vi "AllAvrStdGraph.vi"() -> ()   [LabVIEW 2023]
panel:
  out "Numeric":dbl format="%#_4f"
  out "AvrSTDToArr - only six":dbl[](array[numeric]) format="%#_6f"
  out "Waveform Graph":dbl[][](graph)
  in  "const + StdAvr":dbl
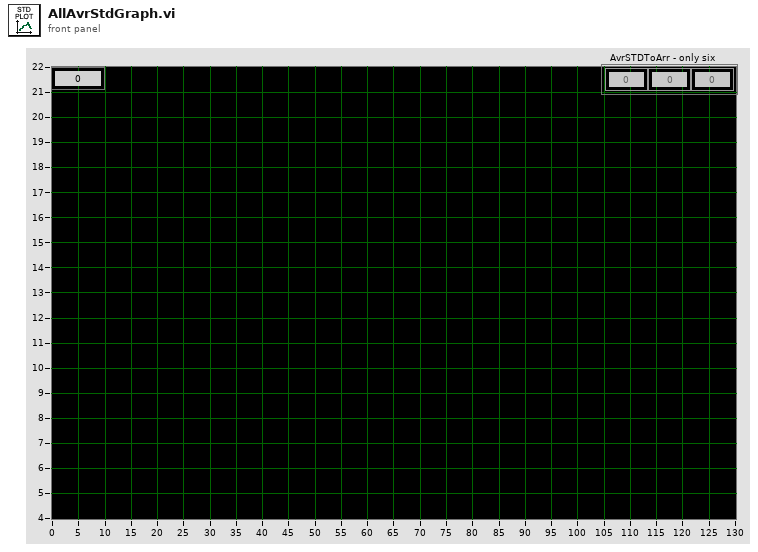
[diagram p1: front panel]
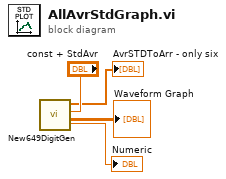
[diagram p0: block diagram]
diagram:
  n1 = call "New649DigitGen.vi"("const + StdAvr"="const + StdAvr") -> ("Waveform Graph"=→"Waveform Graph":dbl[][], "CurrAvrSTDToArr - only six"=→"AvrSTDToArr - only six":dbl[], "lastStd"=→"Numeric":dbl)  [unwired: 7 in, 1 out]
